vi "Do.vi"(8 "error in (no error)":errorcluster, 10 "Actor in":refnum<class "Actor.lvclass">, 11 "Arm Msg":refnum<class "Arm Msg.lvclass">) -> (0 "error out":errorcluster, 2 "Actor out":refnum<class "Actor.lvclass">)   [LabVIEW 2021, in "Arm Msg.lvclass"]
doc: "This VI delivers the message to the actor by calling the appropriate method(s) on the actor."
uses:
  Arm Msg.lvclass
  Arm Msg.lvclass/Arm Msg.ctl
  c61e4209-a6ad-4187-9474-07425d0ed6b0.vi
  Pulse Recorder/Pulse Recorder.lvclass
  <vilib>/ActorFramework/Actor/Actor.lvclass
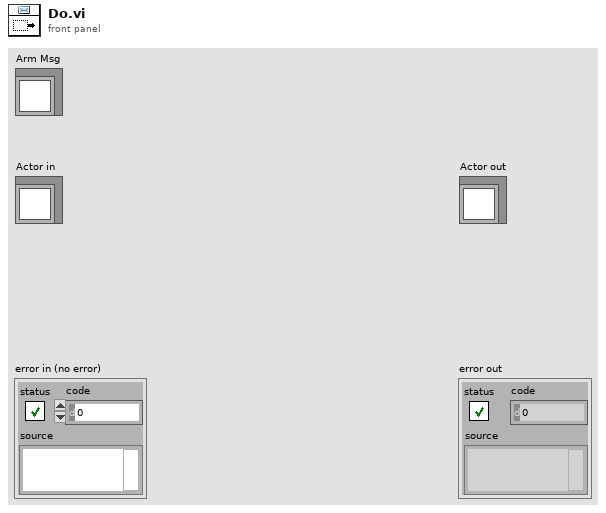
[diagram p1: front panel]
types:
  T1 = typedef "Request type.ctl" = enum16{"Process complete", "User command", "Auto-restart", "Error"}
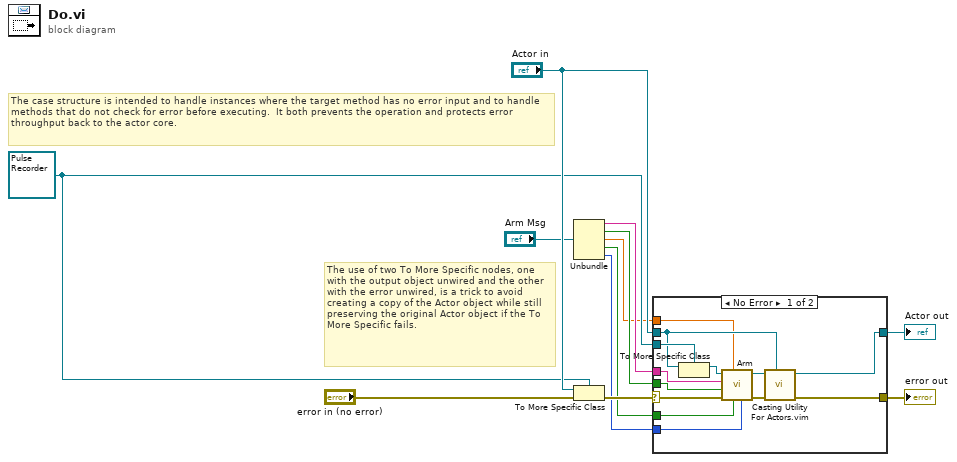
[diagram p0: block diagram]
diagram:
  w7 = refnum<class "Pulse Recorder.lvclass"> refnum ("Actor in")
  # "The use of two To More Specific nodes, one with the output object unwired and the other with the error unwired, is a trick to avoid creating a copy of the Actor object while still preserving the original Actor object if the To More Specific fails."
  # "The case structure is intended to handle instances where the target method has no error input and to handle methods that do not check for error before executing.  It both prevents the operation and protects error throughput back to the actor core."
  n1 = Unbundle("Arm Msg") -> (w5:string, w4:bool, w3:dbl, w2:bool, w1:T1)
  n2 = To More Specific Class(target class=w7, reference="Actor in", error in="error in (no error)") -> (error out=w6:errorcluster)  [unwired: 1 out]
  n3 = case shown="No Error" w6 {
    selector: w6 -> [w25 w27]
    tunnel: [w19 w27] -> w12
    tunnel: [w20 w26] -> w11
    tunnel: "Actor in" -> [w22 w26]
    tunnel: w7 -> [w23 _]
    tunnel: w5 -> [w17 _]
    tunnel: w4 -> [w16 _]
    tunnel: w3 -> [w15 _]
    tunnel: w2 -> [w14 _]
    tunnel: w1 -> [w13 _]
    frame No Error {
      n4 = To More Specific Class(target class=w23, reference=w22) -> (specific class reference=w24:refnum<class "Pulse Recorder.lvclass">)  [unwired: 1 in, 1 out]
      n5 = call-dynamic "Arm.vi"("Request type"=w13, "Init work"=w14, "Update period"=w15, "error in (no error)"=w25, "Last request"=w16, "Requester"=w17, "Pulse Recorder in"=w24) -> ("error out"=w18:errorcluster, "Pulse Recorder out"=w21:refnum<class "Pulse Recorder.lvclass">)  [unwired: 3 in]
      n6 = call "Casting Utility For Actors.vim"("type"=w22, "error in (no error)"=w18, "Actor in"=w21) -> ("error out"=w19:errorcluster, "Actor out"=w20:refnum<class "Actor.lvclass">)  [unwired: 7 in]
    }
    frame Error {
      # "If type check fails, pass the original object out again."
    }
  }
  "error out" <- w12
  "Actor out" <- w11
